vi "launch target selector.vi"(8 "error in (no error)":errorcluster, 10 "Options":string[](array[string])) -> (0 "error out":errorcluster, 1 "Canceled?":bool, 3 "Target Index":i32)   [LabVIEW 2013, in "Standard Editor.lvlib"]
uses:
  Standard Editor.lvlib
  target selector.vi
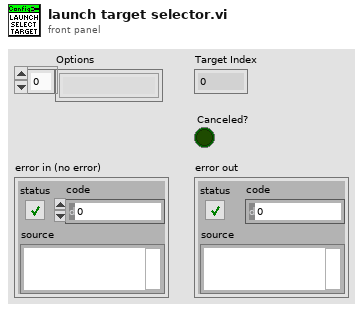
[diagram p1: front panel]
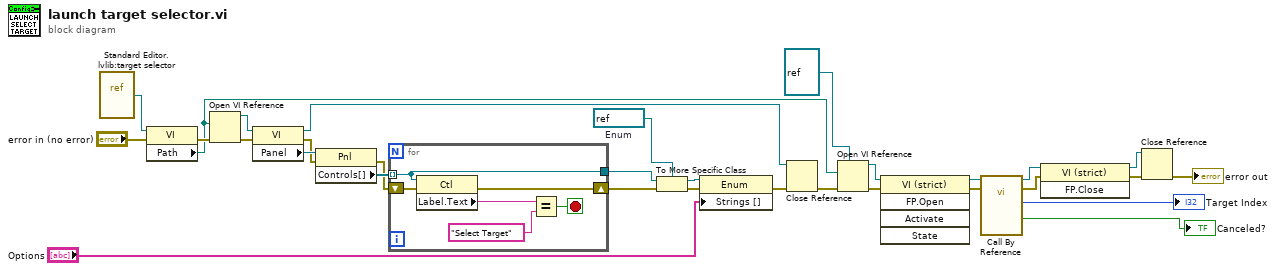
[diagram p0: block diagram]
diagram:
  w26 = refnum<vi> refnum  # Enum
  n1 = vi-ref "Standard Editor.lvlib:target selector.vi"() -> (w31:refnum<vi>)
  n2 = property class="VI"(reference=w31, error in="error in (no error)") -> (error out=w22:errorcluster, "Path"=w9:path)  [unwired: 1 out]
  n3 = Open VI Reference(vi path=w9, error in (no error)=w22) -> (vi reference=w30:refnum<vi>, error out=w21:errorcluster)  [unwired: 4 in]
  n4 = property class="VI"(reference=w30, error in=w21) -> (reference out=w10:refnum<vi>, error out=w20:errorcluster, "Panel"=w29:refnum<vi>)
  n5 = property class="Pnl"(reference=w29, error in=w20) -> (error out=w19:errorcluster, "Controls[]"=w28:refnum<vi>[])  [unwired: 1 out]
  n6 = for {
    tunnel: w28 -> [w35] mode=indexing
    tunnel: [w35] -> w27
    shift-right: [w32] -> w18
    shift-left: w19 -> [w33]
    stop <- w34 stop-if-true
    n7 = property class="Ctl"(reference=w35, error in=w33) -> (error out=w32:errorcluster, "Label.Text"=w37:string)  [unwired: 1 out]
    n8 = Equal?(x=w37, y="Select Target") -> (x = y?=w34:bool)
  }
  n9 = To More Specific Class(target class=w26, reference=w27, error in=w18) -> (specific class reference=w25:refnum<vi>, error out=w23:errorcluster)
  n10 = property class="Enum"(reference=w25, error in=w23, "Strings []"="Options") -> (error out=w6:errorcluster)  [unwired: 1 out]
  n11 = Close Reference(reference=w10, error in (no error)=w6) -> (error out=w5:errorcluster)
  n12 = Open VI Reference(type specifier VI Refnum (for type only)=refnum<vi> refnum, vi path=w9, error in (no error)=w5) -> (vi reference=w8:refnum<vi>, error out=w7:errorcluster)  [unwired: 3 in]
  n13 = invoke class="VI (strict)" method="FP.Open"(reference=w8, error in=w7) -> (reference out=w16:refnum<vi>, error out=w12:errorcluster)  [unwired: 3 in, 3 out]
  n14 = call-by-ref "?"(reference=w16, error in=w12) -> (reference out=w15:refnum<vi>, error out=w13:errorcluster, "Canceled?"=→"Canceled?":bool, "Target Index"=→"Target Index":i32)  [unwired: 10 in]
  n15 = invoke class="VI (strict)" method="FP.Close"(reference=w15, error in=w13) -> (reference out=w3:refnum<vi>, error out=w2:errorcluster)  [unwired: 1 in, 1 out]
  n16 = Close Reference(reference=w3, error in (no error)=w2) -> (error out=→"error out":errorcluster)
